vi "_TEST.Simple TCP-IP Sender.vi"() -> ()   [LabVIEW 2016]
panel:
  in  "Send":bool
  in  "String":string
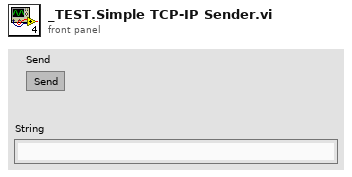
[diagram p1: front panel]
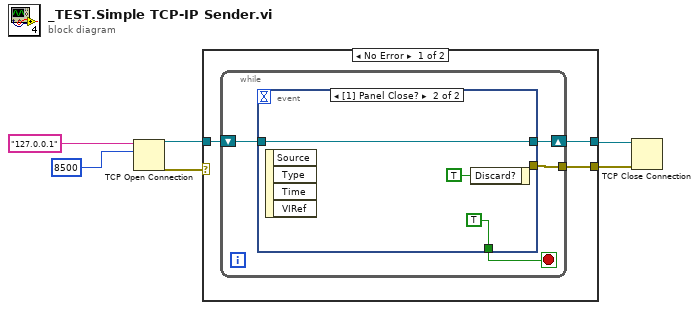
[diagram p0: block diagram]
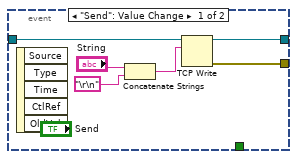
[diagram p2: hidden frame]
diagram:
  n1 = TCP Open Connection(address="127.0.0.1", remote port or service name=u16 8500) -> (connection ID=w4:refnum<k5>, error out=w3:errorcluster)  [unwired: 3 in]
  n2 = case shown="No Error" w3 {
    tunnel: w4 -> [w9 w23]
    tunnel: [w8 w23] -> w2
    tunnel: [w7 _] -> w1
    frame No Error {
      n3 = while {
        shift-right: [w12] -> w8
        shift-left: w9 -> [w13]
        tunnel: [w11] -> w7
        stop <- w10 stop-if-true
        n4 = event shown="[1] Panel Close?" {
          selector: _ -> [_ _]
          dyn-events: _ -> [_ _]
          timeout: _ -> [_ _]
          tunnel: w13 -> [w19 w21]
          tunnel: [w18 w21] -> w12
          tunnel: [w17 _] -> w11
          tunnel: [_ TRUE] -> w10
          event "Send": Value Change {
            n5 = event-data() -> ()  [unwired: 1 in, 5 out]
            n6 = Concatenate Strings("String", "\r\n") -> (w14:string)
            n7 = TCP Write(connection ID=w19, data in=w14) -> (connection ID out=w18:refnum<k5>, error out=w17:errorcluster)  [unwired: 2 in, 1 out]
          }
          event Panel Close? {
            n8 = event-data() -> ()  [unwired: 1 in, 4 out]
            n9 = event-data("Discard?"=TRUE) -> ()  [unwired: 1 in, 1 out]
          }
        }
      }
    }
    frame Error {
    }
  }
  n10 = TCP Close Connection(connection ID=w2, error in (no error)=w1) -> ()  [unwired: 1 in, 2 out]
